vi "Save all VIs in Folder.vi"() -> ()   [LabVIEW 2021]
panel:
  out "total":i32
  out "open":i32
  out "save":i32
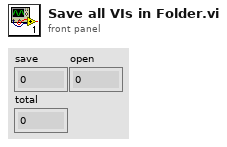
[diagram p1: front panel]
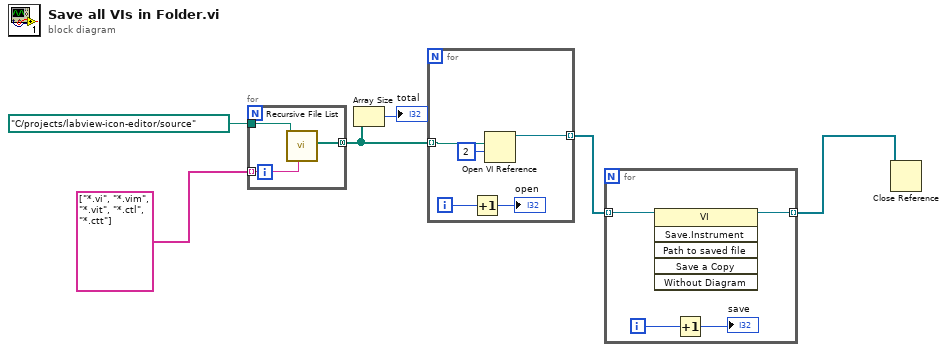
[diagram p0: block diagram]
diagram:
  n1 = for {
    tunnel: path "C:/projects/labview-icon-editor/source" -> [w9]
    tunnel: string[] ["*.vi", "*.vim", "*.vit", "*.ctl", "*.ctt"] -> [w8] mode=indexing
    tunnel: [w7] -> w3 mode=concatenating
    n2 = call <vilib>:"Recursive File List.vi"("pattern"=w8, "Folder Path"=w9) -> ("All Files in Dir"=w7:path[])  [unwired: 5 in, 4 out]
  }
  n3 = Array Size(array=w3) -> (size(s)=→"total":i32)
  n4 = for {
    tunnel: w3 -> [w14] mode=indexing
    tunnel: [w13] -> w5 mode=indexing
    i -> [w12]
    n5 = Increment(x=w12) -> (x+1=→"open":i32)
    n6 = Open VI Reference(vi path=w14, options=2) -> (vi reference=w13:refnum<vi>)  [unwired: 4 in, 1 out]
  }
  n7 = for {
    tunnel: w5 -> [w18] mode=indexing
    tunnel: [w17] -> w4 mode=indexing
    i -> [w16]
    n8 = invoke class="VI" method="Save.Instrument"(reference=w18) -> (reference out=w17:refnum<vi>)  [unwired: 5 in, 5 out]
    n9 = Increment(x=w16) -> (x+1=→"save":i32)
  }
  n10 = Close Reference(reference=w4) -> ()  [unwired: 1 in, 1 out]
